vi "Init.vi"(8 "error in (no error)":errorcluster, 11 "Report Generator In":refnum<class "Report Generator.lvclass">) -> (0 "error out":errorcluster, 3 "Report Generator Out":refnum<class "Report Generator.lvclass">)   [LabVIEW 2020, in "Report Generation.lvlib" / "Report Generator.lvclass"]
uses:
  Report Generator.lvclass
  Report Generator.vi
  User Interface/Process/Process.lvclass
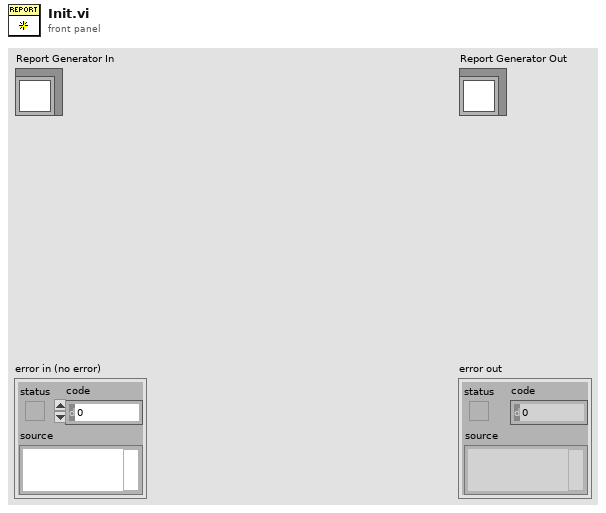
[diagram p1: front panel]
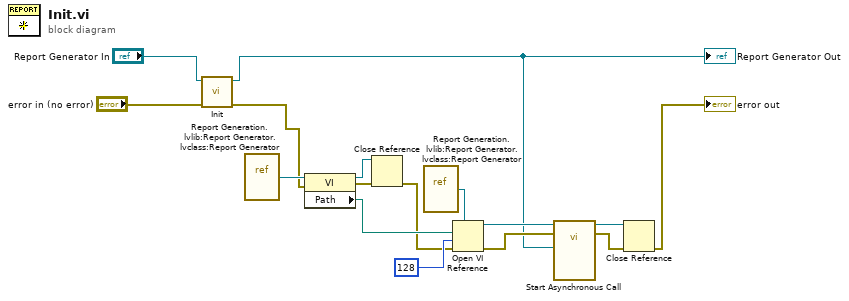
[diagram p0: block diagram]
diagram:
  n1 = call-parent "Init.vi"("error in (no error)"="error in (no error)", "Process In"="Report Generator In") -> ("error out"=w3:errorcluster, "Process Out"=w1:refnum<class "Report Generator.lvclass">)  [unwired: 8 in]
  "Report Generator Out" <- w1
  n2 = vi-ref "Report Generation.lvlib:Report Generator.lvclass:Report Generator.vi"() -> (w14:refnum<vi>)
  n3 = property class="VI"(reference=w14, error in=w3) -> (reference out=w4:refnum<vi>, error out=w7:errorcluster, "Path"=w12:path)
  n4 = Close Reference(reference=w4, error in (no error)=w7) -> (error out=w6:errorcluster)
  n5 = vi-ref "Report Generation.lvlib:Report Generator.lvclass:Report Generator.vi"() -> (w13:refnum<vi>)
  n6 = Open VI Reference(type specifier VI Refnum (for type only)=w13, vi path=w12, options=128, error in (no error)=w6) -> (vi reference=w10:refnum<vi>, error out=w5:errorcluster)  [unwired: 2 in]
  n7 = call-by-ref "Start Asynchronous Call"(reference=w10, error in=w5, "Report Generator In"=w1) -> (reference out=w9:refnum<vi>, error out=w8:errorcluster)  [unwired: 10 in, 1 out]
  n8 = Close Reference(reference=w9, error in (no error)=w8) -> (error out=→"error out":errorcluster)
